vi "Pre Launch Init.vi"(11 "Actor_Log in":refnum<class "Actor_EventStart.lvclass">) -> (0 "error out":errorcluster, 3 "Actor_Log out":refnum<class "Actor_EventStart.lvclass">)   [LabVIEW 2020, in "Library Core.lvlib" / "Actor_EventStart.lvlib" / "Actor_EventStart.lvclass"]
doc: "(<B>Filename</B>: Actor Framework.lvlib:Actor.lvclass:Pre Launch Init.vi)\n\nDefines behavior that occurs after the Launch Nested Actor method is invoked but before the actor's Actor Core method begins running.\n\nBy default, this method does nothing. A descendant class may override it to define behavior."
uses:
  Actor_EventStart.lvclass
  C:/Program Files (x86)/National Instruments/LabVIEW 2020/vi.lib/ActorFramework/Actor/Actor.lvclass
  <vilib>/ActorFramework/Actor/Actor.lvclass/Actor.ctl
  <vilib>/ActorFramework/Message Enqueuer/Message Enqueuer.lvclass/Message Enqueuer.ctl
  Actor_EventStart.lvclass/Actor_EventStart.ctl
  Actor_EventStart Messages/Message Show_GUI/Message Show_GUI.lvclass/Message Show_GUI.ctl
  Actor_EventStart Messages/Message State/Message State.lvclass/Message State.ctl
  <vilib>/ActorFramework/Message Enqueuer/Init from Existing Queue.vi
  <vilib>/ActorFramework/Message Enqueuer/Enqueue.vi
  <vilib>/ActorFramework/Stop Msg/Stop Msg.lvclass
  C:/Program Files (x86)/National Instruments/LabVIEW 2020/vi.lib/ActorFramework/Message/Message.lvclass
  Actor_EventStart Messages/Message Show_GUI/Message Show_GUI.lvclass
  Actor_EventStart Messages/Message State/Message State.lvclass
  <vilib>/ActorFramework/Message Priority Queue/Priority Enqueue.vi
  <vilib>/ActorFramework/Message Enqueuer/Message Enqueuer.lvclass
  <vilib>/ActorFramework/Actor/Actor.lvclass
  Commun VI/Library Commun.lvlib
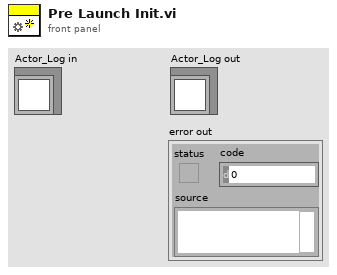
[diagram p1: front panel]
types:
  T1 = enum16{"Init", "Add Actor", "Delete Actor", "Get Actor Queue", "Get Log Actor Queue", "List all actors"}
  T2 = enum16{"Not Use", "Wait Event", "Test in progress", "Test Stopped"}
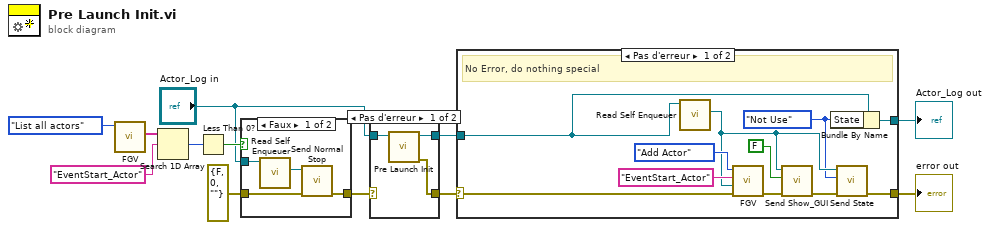
[diagram p0: block diagram]
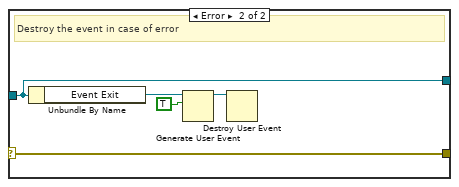
[diagram p3: hidden frame]
diagram:
  n1 = call "FGV.vi"("Action"=T1."List all actors") -> ("Actor names"=w7:string[])  [unwired: 8 in, 2 out]
  n2 = Search 1D Array(1D array=w7, element="EventStart_Actor") -> (index of element=w5:i32)  [unwired: 1 in]
  n3 = Less Than 0?(x=w5) -> (x < 0?=w3:bool)
  n4 = case shown="Faux" w3 {
    tunnel: "Actor_Log in" -> [w16 _]
    tunnel: errorcluster {"status"=FALSE, "code"=0, "source"=""} ("error out") -> [w14 w17]
    tunnel: [w13 w17] -> w4
    frame False {
      n5 = call <vilib>:"Read Self Enqueuer.vi"("Actor"=w16) -> ("Self Enqueuer"=w15:refnum<class "Message Enqueuer.lvclass">)  [unwired: 10 in]
      n6 = call <vilib>:"Send Normal Stop.vi"("error in (no error)"=w14, "Message Enqueuer"=w15) -> ("error out"=w13:errorcluster)  [unwired: 9 in]
    }
    frame True {
    }
  }
  n7 = case shown="Pas d'erreur" w4 {
    selector: w4 -> [_ w22]
    tunnel: [w20 w22] -> w12
    tunnel: "Actor_Log in" -> [w19 w21]
    tunnel: [w18 w21] -> w11
    frame No Error {
      n8 = call-parent "Pre Launch Init.vi"("Actor in"=w19) -> ("error out"=w20:errorcluster, "Actor out"=w18:refnum<class "Actor_EventStart.lvclass">)  [unwired: 9 in]
    }
    frame Error {
    }
  }
  n9 = case shown="Pas d'erreur" w12 {
    selector: w12 -> [w32 w34]
    tunnel: w11 -> [w30 w35]
    tunnel: [w26 w34] -> w10
    tunnel: [w29 w35] -> w9
    frame No Error {
      w24 = T2."Not Use" ("State")
      # "No Error, do nothing special"
      n10 = call <vilib>:"Read Self Enqueuer.vi"("Actor"=w30) -> ("Self Enqueuer"=w25:refnum<class "Message Enqueuer.lvclass">)  [unwired: 10 in]
      n11 = call "FGV.vi"("error in (no error)"=w32, "Actor's Queue In"=w25, "Actor name"="EventStart_Actor", "Action"=T1."Add Actor") -> ("error out"=w28:errorcluster)  [unwired: 5 in, 2 out]
      n12 = call "Send Show_GUI.vi"("error in (no error)"=w28, "Show_GUI"=FALSE, "Message Enqueuer"=w25) -> ("error out"=w27:errorcluster)  [unwired: 7 in, 1 out]
      n13 = Bundle By Name(cluster=w30, "State"=w24) -> (w29:refnum<class "Actor_EventStart.lvclass">)
      n14 = call "Send State.vi"("error in (no error)"=w27, "State"=w24, "Message Enqueuer"=w25) -> ("error out"=w26:errorcluster)  [unwired: 7 in, 1 out]
    }
    frame Error {
      # "Destroy the event in case of error"
      n15 = Unbundle By Name(w35) -> ("Event Exit"=w38:refnum<user-event>)
      n16 = Generate User Event(user event=w38, event data cluster=TRUE ("event data")) -> (user event out=w36:refnum<user-event>)  [unwired: 2 in, 1 out]
      n17 = Destroy User Event(user event=w36) -> ()  [unwired: 1 in, 1 out]
    }
  }
  "error out" <- w10
  "Actor_Log out" <- w9
